vi "NF WF1973_74 OFSM.vi"(6 "Read(F)":bool, 7 "Deviation(0)":dbl min=0.0 max=10.0 step=0.0001 format="%.4f", 8 "error in (no error)":errorcluster caption="Error IN", 9 "Set Deviation(Input)":u16(ring) items=["Input", "Minimum", "Maximum"], 10 "Ch(Ch1)":bool, 11 "VISAsession":refnum<visa-resource-name>) -> (0 "error out":errorcluster caption="Error OUT", 2 "Query Deviation":dbl=9999.0 format="%.4f", 3 "CopyVISAsession":refnum<visa-resource-name>)   [LabVIEW 2010]
panel:
  in  "Units(V)":u16(ring)=1 items=["mV", "V"]
  # "Choose\nInput"
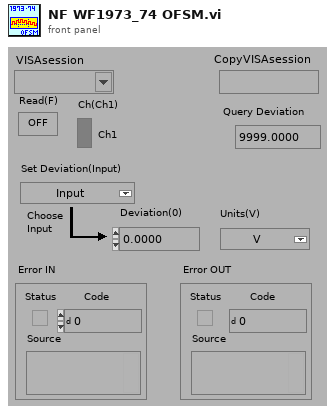
[diagram p1: front panel]
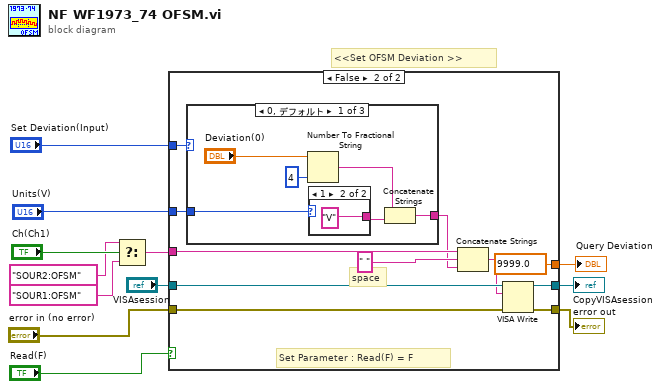
[diagram p0: block diagram]
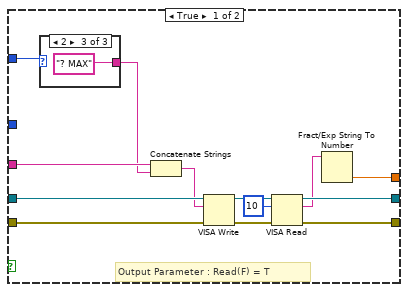
[diagram p2: hidden frame]
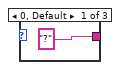
[diagram p3: hidden frame]
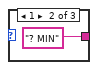
[diagram p4: hidden frame]
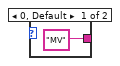
[diagram p5: hidden frame]
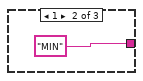
[diagram p6: hidden frame]
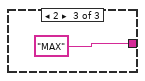
[diagram p7: hidden frame]
diagram:
  # "<<Set OFSM Deviation >>"
  n1 = Select(t="SOUR2:OFSM" ("文字列"), s="Ch(Ch1)", f="SOUR1:OFSM" ("文字列")) -> (s? t:f=w5:string)
  n2 = case shown="FALSE" "Read(F)" {
    tunnel: "VISAsession" -> [w25 w39]
    tunnel: [w22 w37] -> w11
    tunnel: [w21 w38] -> w10
    tunnel: "error in (no error)" -> [w20 w33]
    tunnel: w5 -> [w18 w34]
    tunnel: [w15 9999.0] -> w7
    tunnel: "Set Deviation(Input)" -> [w14 w32]
    tunnel: "Units(V)" -> [_ w29]
    frame True {
      # "Output Parameter : Read(F) = T"
      n3 = case shown="2" w14 {
        tunnel: ["?" ("形式文字列") "? MIN" ("形式文字列") "? MAX" ("形式文字列")] -> w13
        frame 0, Default {
        }
        frame 1 {
        }
        frame 2 {
        }
      }
      n4 = Concatenate Strings(w18, w13) -> (w17:string)
      n5 = VISA Write(VISA resource name=w25, write buffer=w17, error in (no error)=w20) -> (VISA resource name out=w23:refnum<visa-resource-name>, error out=w24:errorcluster)  [unwired: 1 out]
      n6 = VISA Read(VISA resource name=w23, byte count=u32 10 ("バイトカウント（0）"), error in (no error)=w24) -> (VISA resource name out=w22:refnum<visa-resource-name>, read buffer=w16:string, error out=w21:errorcluster)  [unwired: 1 out]
      n7 = Fract/Exp String To Number(string=w16) -> (number=w15:dbl)  [unwired: 3 in, 1 out]
    }
    frame False {
      # "space"
      # "Set Parameter : Read(F) = F"
      n8 = case shown="0, デフォルト" w32 {
        tunnel: [w45 "MIN" ("文字列") "MAX" ("文字列")] -> w31
        tunnel: w29 -> [w40 _ _]
        frame 0, Default {
          n9 = Number To Fractional String(number="Deviation(0)", precision (6)=i16 4 ("精度 (6)")) -> (F-format string=w42:string)  [unwired: 2 in]
          n10 = case shown="1" w40 {
            tunnel: ["MV" "V"] -> w41
            frame 0, Default {
            }
            frame 1 {
            }
          }
          n11 = Concatenate Strings(w42, w41) -> (w45:string)
        }
        frame 1 {
        }
        frame 2 {
        }
      }
      n12 = Concatenate Strings(w34, " ", w31) -> (w36:string)
      n13 = VISA Write(VISA resource name=w39, write buffer=w36, error in (no error)=w33) -> (VISA resource name out=w37:refnum<visa-resource-name>, error out=w38:errorcluster)  [unwired: 1 out]
    }
  }
  "error out" <- w10
  "CopyVISAsession" <- w11
  "Query Deviation" <- w7
